vi "Instrument Do Core.vi"(8 "error in (no error)":errorcluster, 9 "Instrument in":refnum<class "Instrument Driver.lvclass">, 10 "Actor in":refnum<class "Actor.lvclass">, 11 "DMM Immediate Measure Msg in":refnum<class "DMM Immediate Measure Msg.lvclass">) -> (0 "error out":errorcluster, 1 "Instrument out":refnum<class "Instrument Driver.lvclass">, 2 "Actor out":refnum<class "Actor.lvclass">, 3 "DMM Immediate Measure Msg out":refnum<class "DMM Immediate Measure Msg.lvclass">, 5 "Data":refnum<class "Data.lvclass">)   [LabVIEW 2020, in "DMM Msg.lvlib" / "DMM Immediate Measure Msg.lvclass"]
doc: "Perform a measurement using the DMM and returning the results in a DMM Measurement Data class."
uses:
  DMM Immediate Measure Msg.lvclass
  PPL/HDH.Actor Framework.Core.Actor.lvlibp/1abvi3w/vi.lib/ActorFramework/Actor/Actor.lvclass
  PPL/HDH.Data.Generic.lvlibp/Data.lvclass
  PPL/HDH.Actor Framework.Core.Instrument Driver.lvlibp/Instrument Driver/Instrument Driver.lvclass
  PPL/HDH.Driver.DMM.lvlibp/DMM Driver.lvclass
  C:/Current projects/WS/PPL/HDH.Actor Framework.Core.Instrument Driver.lvlibp/Instrument Driver/Instrument Driver.lvclass
  Data/DMM Measurement Data/DMM Measurement Data.lvclass
  C:/Current projects/WS/PPL/HDH.Data.Generic.lvlibp/Data.lvclass
  DMM Immediate Measure Msg.lvclass/DMM Immediate Measure Msg.ctl
  Data/DMM Measurement Data/DMM Measurement Data.lvclass/DMM Measurement Data.ctl
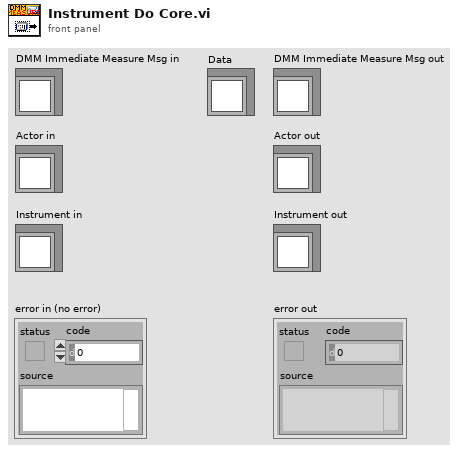
[diagram p1: front panel]
types:
  T1 = typedef "HDH.Driver.DMM.lvlibp/Ctl_Function.ctl" = enum8{"DC Volts", "AC Volts", "DC Current", "AC Current", "2-wire Resistance", "4-wire Resistance", "Diode", "Frequency", "Period", "AC Volts DC Coupled", "Capacitance", "Inductance", "Temperature"}
  T2 = typedef "HDH.Driver.DMM.lvlibp/Ctl_DigitResolution.ctl" = enum8{"3½", "4½", "5½", "6½", "7½"}
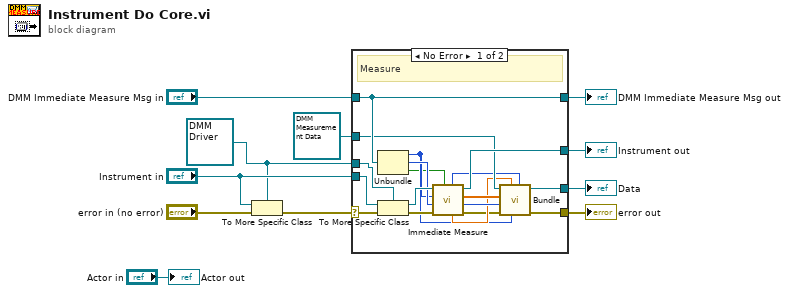
[diagram p0: block diagram]
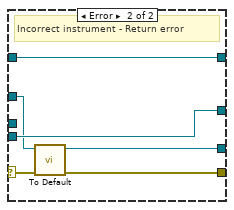
[diagram p2: hidden frame]
diagram:
  w5 = refnum<class "DMM Driver.lvclass"> refnum ("HDH.Driver.DMM.lvlibp:DMM Driver.lvclass")
  n1 = To More Specific Class(target class=w5, reference="Instrument in", error in="error in (no error)") -> (error out=w10:errorcluster)  [unwired: 1 out]
  n2 = case shown="No Error" w10 {
    selector: w10 -> [w29 w31]
    tunnel: [w13 w30] -> w3
    tunnel: [w26 w35] -> w9
    tunnel: "DMM Immediate Measure Msg in" -> [w26 w35]
    tunnel: [w23 w34] -> w7
    tunnel: "Instrument in" -> [w28 w34]
    tunnel: w5 -> [w27 _]
    tunnel: [w20 w32] -> w2
    tunnel: refnum<class "DMM Measurement Data.lvclass"> refnum ("DMM Measurement Data in") -> [w21 w33]
    frame No Error {
      # "Measure"
      n3 = Unbundle(w26) -> (w15:i32, w22:i32, w12:bool)
      n4 = To More Specific Class(target class=w27, reference=w28, error in=w29) -> (specific class reference=w24:refnum<class "DMM Driver.lvclass">, error out=w25:errorcluster)
      n5 = call "Immediate Measure.vi"("Restore Range?(T)"=w12, "error in (no error)"=w25, "Max Time (-1ms)"=w22, "Measurements to Acquire(1)"=w15, "DMM Driver in"=w24) -> ("error out"=w14:errorcluster, "Function"=w17:T1, "Measurements"=w18:dbl[], "DMM Driver out"=w23:refnum<class "DMM Driver.lvclass">, "Range"=w16:dbl, "Digit Resolution(5½)"=w19:T2)  [unwired: 1 in]
      n6 = call "Bundle.vi"("Digit Resolution"=w19, "Target Measurement Count"=w15, "Range"=w16, "error in (no error)"=w14, "Function"=w17, "Measurements"=w18, "DMM Measurement Data in"=w21) -> ("error out"=w13:errorcluster, "DMM Measurement Data out"=w20:refnum<class "DMM Measurement Data.lvclass">)  [unwired: 3 in]
    }
    frame Error {
      # "Incorrect instrument - Return error"
      n7 = call-dynamic "To Default.vi"("error in (no error)"=w31, "Data in"=w33) -> ("error dub"=w30:errorcluster, "Data out"=w32:refnum<class "DMM Measurement Data.lvclass">)  [unwired: 8 in]
    }
  }
  "error out" <- w3
  "DMM Immediate Measure Msg out" <- w9
  "Instrument out" <- w7
  "Data" <- w2
  "Actor out" <- "Actor in"
